vi "Drive SSS.vi"(11 "Drive SS Actuator Values In":T1) -> (3 "Drive SS Actuator Values Out":T1)   [LabVIEW 2014]
uses:
  Drive SS Actuator Values.ctl
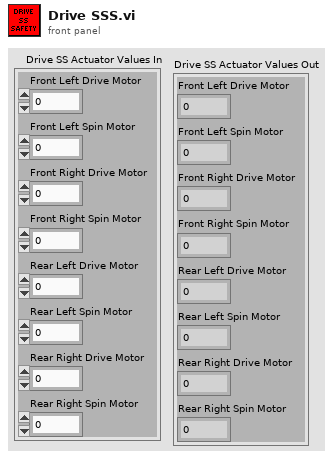
[diagram p1: front panel]
types:
  T1 = typedef "Drive SS Actuator Values.ctl" = cluster{"Front Left Drive Motor":dbl, "Front Left Spin Motor":dbl, "Front Right Drive Motor":dbl, "Front Right Spin Motor":dbl, "Rear Left Drive Motor":dbl, "Rear Left Spin Motor":dbl, "Rear Right Drive Motor":dbl, "Rear Right Spin Motor":dbl}
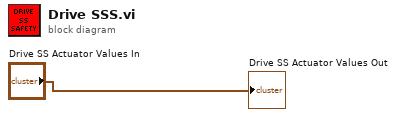
[diagram p0: block diagram]
diagram:
  "Drive SS Actuator Values Out" <- "Drive SS Actuator Values In"
